vi "Write Dispatcher Error.vi"(8 "error in (no error)":errorcluster, 9 "timeout in ms (0)":i32 format="%d ms", 10 "error":errorcluster, 11 "Dispatcher Interface in":refnum<class "Dispatcher Interface.lvclass">) -> (0 "error out":errorcluster, 3 "Dispatcher Interface out":refnum<class "Dispatcher Interface.lvclass">)   [LabVIEW 2017, in "DSF Core.lvlib" / "Dispatcher Interface.lvclass"]
uses:
  Dispatcher Interface.lvclass
  C:/Users/Admin/Desktop/Data Sharing Framework/Source/Core/Engine/Classes/Interfaces/Interface/Interface.lvclass
  Interface/Interface.lvclass/Interface.ctl
  Interface/Write Error Queue.vi
  Error Timeout.vi
  Interface/Interface.lvclass
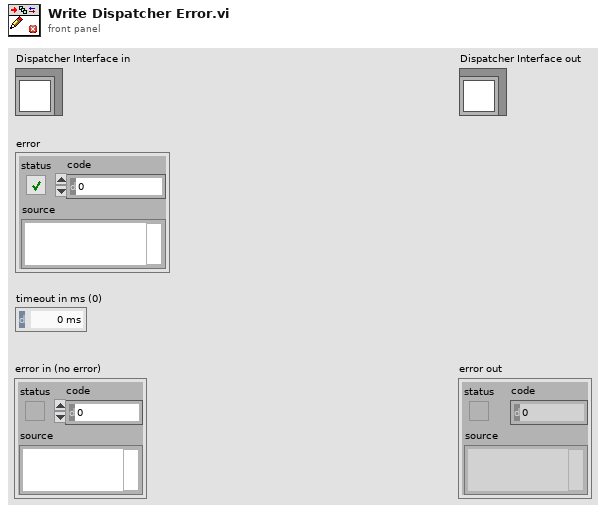
[diagram p1: front panel]
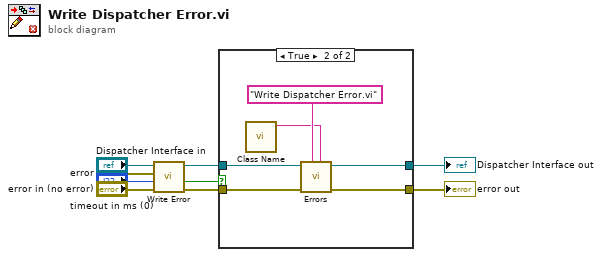
[diagram p0: block diagram]
diagram:
  n1 = call "Write Error.vi"("error in (no error)"="error in (no error)", "timeout in ms (0)"="timeout in ms (0)", "error"="error", "Interface in"="Dispatcher Interface in") -> ("error out"=w4:errorcluster, "timed out?"=w3:bool, "Interface out"=w5:refnum<class "Dispatcher Interface.lvclass">)  [unwired: 5 in]
  n2 = case shown="True" w3 {
    tunnel: w4 -> [w10 w15]
    tunnel: w5 -> [w11 w16]
    tunnel: [w11 w14] -> w2
    tunnel: [w10 w13] -> w1
    frame False {
    }
    frame True {
      n3 = call "Class Name.vi"() -> ("class name"=w12:string)  [unwired: 11 in]
      n4 = call-poly "Errors.vi"("error source class name"=w12, "error source vi name"="Write Dispatcher Error.vi", "error in (no error)"=w15, "Interface in"=w16) -> ("error out"=w13:errorcluster, "Interface out"=w14:refnum<class "Dispatcher Interface.lvclass">)  [unwired: 6 in]
    }
  }
  "error out" <- w1
  "Dispatcher Interface out" <- w2
